vi "LabelEncoder.vi"(8 "error in (no error)":errorcluster caption="entrée d'erreur (pas d'erreur)") -> (0 "error out":errorcluster, 3 "LabelEncoder.lvclass":refnum<class "LabelEncoder.lvclass">)   [LabVIEW 2020]
doc: "Encode target labels with value between 0 and n_classes-1.\n\nThis transformer should be used to encode target values, i.e. y, and not the input X.\n\n\nMethods : \n\n\n- Fit : Fit label encoder\n\nParameters : y : array-like of shape (n_samples,)\n Target values.\n\n- Fit Transform : Fit label encoder and return encoded labels\n\nParameters : y : array-like of shape [n_samples]\n Target values.\n\nReturns : y : array-like of shape [n_samples]\n\n\n- Transform : Transform labels to normalized encoding.\n\nParameters : y : array-like of shape [n_samples]\n Target values.\n\nReturns : y : array-like of shape [n_samples]"
uses:
  LabelEncoder.lvclass
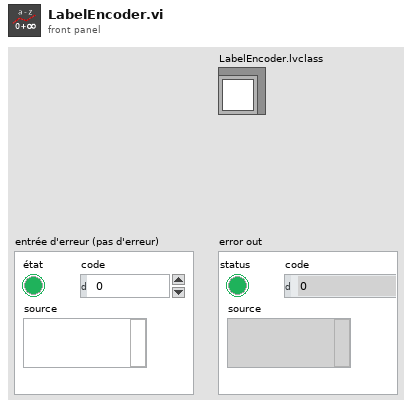
[diagram p1: front panel]
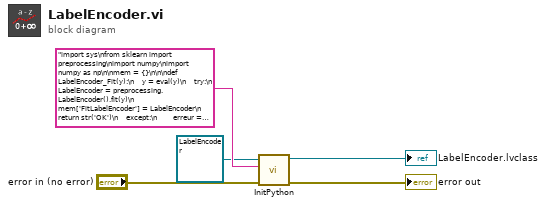
[diagram p0: block diagram]
diagram:
  n1 = call-dynamic "InitPython.vi"("error in (no error)"="error in (no error)", "Python Instruction"="import sys\nfrom sklearn import preprocessing\nimport numpy\nimport numpy as np\n\nmem = {}\n\n\ndef LabelEncoder_Fit(y):\n    y = eval(y)\n    try:\n        LabelEncoder = preprocessing.LabelEncoder().fit(y)\n        mem['FitLabelEncoder'] = LabelEncoder\n        return str('OK')\n    except:\n        erreur = sys.exc_info()\n        typerr = u\"%s\" % (erreur[0])\n        typerr = typerr[typerr.find(\"'\")+1:typerr.rfind(\"'\")]\n        msgerr = u\"%s\" % (erreur[1])\n        message = str('/!\\\\ {0} : {1}'. format(typerr,msgerr))\n        return message \n    \ndef LabelEncoder_FitTransform(y):\n    y = eval(y)\n    try:\n        LabelEncoder = preprocessing.LabelEncoder().fit_transform(y)\n        LabelEncoder = LabelEncoder.tolist()\n        return str(LabelEncoder)\n    except:\n        erreur = sys.exc_info()\n        typerr = u\"%s\" % (erreur[0])\n        typerr = typerr[typerr.find(\"'\")+1:typerr.rfind(\"'\")]\n        msgerr = u\"%s\" % (erreur[1])\n        message = str('/!\\\\ {0} : {1}'. format(typerr,msgerr))\n        return message \n\ndef LabelEncoder_Transform(y):\n    y = eval(y)\n    try:\n        LabelEncoder = mem['FitLabelEncoder'].transform(y)\n        LabelEncoder = LabelEncoder.tolist()\n        return str(LabelEncoder)\n    except:\n        erreur = sys.exc_info()\n        typerr = u\"%s\" % (erreur[0])\n        typerr = typerr[typerr.find(\"'\")+1:typerr.rfind(\"'\")]\n        msgerr = u\"%s\" % (erreur[1])\n        message = str('/!\\\\ {0} : {1}'. format(typerr,msgerr))\n        return message", "Scikit-learn en entrée"=refnum<class "LabelEncoder.lvclass"> refnum ("LabelEncoder.lvclass")) -> ("error out"=→"error out":errorcluster, "Scikit-learn en sortie"=→"LabelEncoder.lvclass":refnum<class "LabelEncoder.lvclass">)  [unwired: 7 in]
